vi "NI_controller_Rel_move.vi"(0 "Initialize":bool, 1 "Velocity (10000)":i32=20000 min=-20000000 max=20000000, 4 "Z  rel (mm)":dbl, 5 "Y rel (mm)":dbl, 6 "Motion System":T2=enum."No Motion Card", 7 "X rel (mm)":dbl, 8 "Motion ID":T3=1 min=1 max=32 step=1) -> (12 "Bd ID Out":T1, 14 "X start (mm)":dbl, 15 "Y start (mm)":dbl, 16 "Z start (mm)":dbl, 17 "X Stop (mm)":dbl, 18 "Y Stop (mm)":dbl, 19 "Z Stop (mm)":dbl)   [LabVIEW 2022 SP3]
uses:
  <vilib>/Motion/FlexMotion/CustomControls/CustomControls.llb/AxisOrVectorSpace To Configure.flx
  <vilib>/Motion/FlexMotion/FunctionsVIs/StartStopMotion.llb/Start Motion (8 axes).flx
  -NI_MotionRoutines/MotionSys.ctl
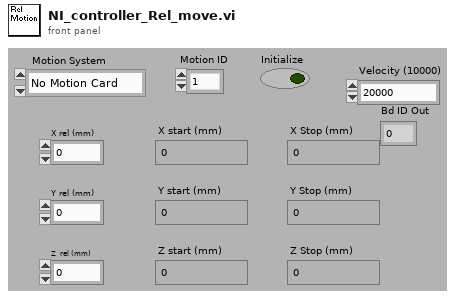
[diagram p1: front panel]
types:
  T1 = typedef "Bd Id Out" = u8
  T2 = typedef "MotionSys.ctl" = enum16{"MM3000", "NI 735x", "Newport ESP", "No Motion Card", "Galil"}
  T3 = typedef "Board Id" = u8
  T4 = enum16{"Absolute Position", "Relative Position", "Velocity", "Relative to Cap Pos", "Modulus Position", "Absolute Contouring", "Relative Contouring"}
  T5 = typedef "AxisOrVectorSpace To Configure.flx" = u16
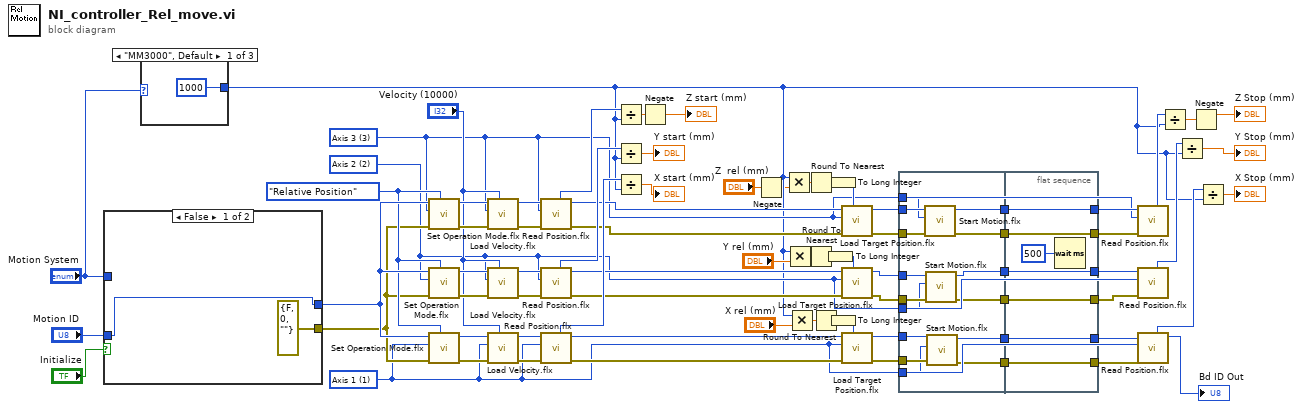
[diagram p0: block diagram]
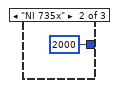
[diagram p2: hidden frame]
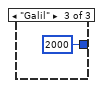
[diagram p3: hidden frame]
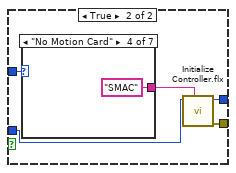
[diagram p4: hidden frame]
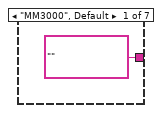
[diagram p5: hidden frame]
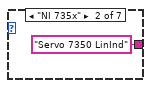
[diagram p6: hidden frame]
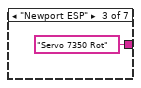
[diagram p7: hidden frame]
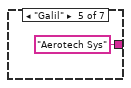
[diagram p8: hidden frame]
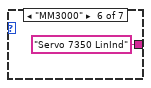
[diagram p9: hidden frame]
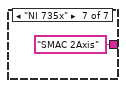
[diagram p10: hidden frame]
diagram:
  w71 = T4."Relative Position" ("Position Mode (Absolute)")
  w18 = T5 3 items=["Axis 1"=1, "Axis 2"=2, "Axis 3"=3, "Axis 4"=4, "Axis 5"=5, "Axis 6"=6, "Axis 7"=7, "Axis 8"=8, "Vector Space 1"=17, "Vector Space 2"=18, "Vector Space 3"=19, "Vector Space 4"=20] ("Axis or Vector Space")
  w19 = T5 2 items=["Axis 1"=1, "Axis 2"=2, "Axis 3"=3, "Axis 4"=4, "Axis 5"=5, "Axis 6"=6, "Axis 7"=7, "Axis 8"=8, "Vector Space 1"=17, "Vector Space 2"=18, "Vector Space 3"=19, "Vector Space 4"=20] ("Axis or Vector Space")
  w17 = T5 1 items=["Axis 1"=1, "Axis 2"=2, "Axis 3"=3, "Axis 4"=4, "Axis 5"=5, "Axis 6"=6, "Axis 7"=7, "Axis 8"=8, "Vector Space 1"=17, "Vector Space 2"=18, "Vector Space 3"=19, "Vector Space 4"=20] ("Axis or Vector Space")
  n1 = case shown="False" "Initialize" {
    tunnel: [w77 w82] -> w72
    tunnel: [errorcluster {"status"=FALSE, "code"=0, "source"=""} ("error out") w81] -> w68
    tunnel: "Motion ID" -> [w77 w79]
    tunnel: "Motion System" -> [_ w78]
    frame False {
    }
    frame True {
      n2 = case shown="\"No Motion Card\"" w78 {
        tunnel: ["" "Servo 7350 LinInd" "Servo 7350 Rot" "SMAC" "Aerotech Sys" "Servo 7350 LinInd" "SMAC 2Axis"] -> w80
        frame "MM3000", Default {
        }
        frame "NI 735x" {
        }
        frame "Newport ESP" {
        }
        frame "No Motion Card" {
        }
        frame "Galil" {
        }
        frame "MM3000" {
        }
        frame "NI 735x" {
        }
      }
      n3 = call <vilib>:"Initialize Controller.flx"("Settings Name"=w80, "Board ID"=w79) -> ("error out"=w81:errorcluster, "Bd ID Out"=w82:T1)  [unwired: 1 in, 5 out]
    }
  }
  n4 = case shown="\"MM3000\", Default" "Motion System" {
    tunnel: [1000 ("y") 2000 ("y") 2000 ("y")] -> w11
    frame "MM3000", Default {
    }
    frame "NI 735x" {
    }
    frame "Galil" {
    }
  }
  n5 = call <vilib>:"Set Operation Mode.flx"("Position Mode (Absolute)"=w71, "error in (no error)"=w68, "Axis or Vector Space"=w18, "Board ID"=w72) -> ("error out"=w67:errorcluster, "Bd ID Out"=w64:T1)  [unwired: 3 out]
  n6 = call <vilib>:"Set Operation Mode.flx"("Position Mode (Absolute)"=w71, "error in (no error)"=w68, "Axis or Vector Space"=w19, "Board ID"=w72) -> ("error out"=w66:errorcluster, "Bd ID Out"=w69:T1)  [unwired: 3 out]
  n7 = call <vilib>:"Set Operation Mode.flx"("Position Mode (Absolute)"=w71, "error in (no error)"=w68, "Axis or Vector Space"=w17, "Board ID"=w72) -> ("error out"=w65:errorcluster, "Bd ID Out"=w70:T1)  [unwired: 3 out]
  n8 = call <vilib>:"Load Velocity.flx"("Velocity (10000)"="Velocity (10000)", "error in (no error)"=w67, "Axis or Vector Space"=w18, "Board ID"=w64) -> ("error out"=w57:errorcluster, "Bd ID Out"=w60:T1)  [unwired: 4 out]
  n9 = call <vilib>:"Load Velocity.flx"("Velocity (10000)"="Velocity (10000)", "error in (no error)"=w66, "Axis or Vector Space"=w19, "Board ID"=w69) -> ("error out"=w58:errorcluster, "Bd ID Out"=w61:T1)  [unwired: 4 out]
  n10 = call <vilib>:"Load Velocity.flx"("Velocity (10000)"="Velocity (10000)", "error in (no error)"=w65, "Axis or Vector Space"=w17, "Board ID"=w70) -> ("error out"=w59:errorcluster, "Bd ID Out"=w62:T1)  [unwired: 4 out]
  n11 = call <vilib>:"Read Position.flx"("error in (no error)"=w57, "Axis"=w18, "Board ID"=w60) -> ("error out"=w47:errorcluster, "Bd ID Out"=w48:T1, "Position"=w54:i32)  [unwired: 4 out]
  n12 = call <vilib>:"Read Position.flx"("error in (no error)"=w58, "Axis"=w19, "Board ID"=w61) -> ("error out"=w46:errorcluster, "Bd ID Out"=w49:T1, "Position"=w55:i32)  [unwired: 4 out]
  n13 = call <vilib>:"Read Position.flx"("error in (no error)"=w59, "Axis"=w17, "Board ID"=w62) -> ("error out"=w45:errorcluster, "Bd ID Out"=w50:T1, "Position"=w56:i32)  [unwired: 4 out]
  n14 = Divide(x=w54, y=w11) -> (x/y=w51:dbl)
  n15 = Divide(x=w55, y=w11) -> (x/y=→"Y start (mm)":dbl)
  n16 = Divide(x=w56, y=w11) -> (x/y=→"X start (mm)":dbl)
  n17 = Negate(x=w51) -> (-x=→"Z start (mm)":dbl)
  n18 = Negate(x="Z  rel (mm)") -> (-x=w10:dbl)
  n19 = Multiply(x=w11, y=w10) -> (x*y=w44:dbl)
  n20 = Multiply(x=w11, y="Y rel (mm)") -> (x*y=w39:dbl)
  n21 = Multiply(x=w11, y="X rel (mm)") -> (x*y=w40:dbl)
  n22 = Round To Nearest(number=w44) -> (nearest integer value=w37:dbl)
  n23 = Round To Nearest(number=w39) -> (nearest integer value=w36:dbl)
  n24 = Round To Nearest(number=w40) -> (nearest integer value=w35:dbl)
  n25 = To Long Integer(number=w36) -> (32bit integer=w33:i32)
  n26 = To Long Integer(number=w37) -> (32bit integer=w34:i32)
  n27 = To Long Integer(number=w35) -> (32bit integer=w32:i32)
  n28 = call <vilib>:"Load Target Position.flx"("Target Position (0)"=w34, "error in (no error)"=w47, "Axis"=w18, "Board ID"=w48) -> ("error out"=w31:errorcluster, "Bd ID Out"=w25:T1)  [unwired: 4 out]
  n29 = call <vilib>:"Load Target Position.flx"("Target Position (0)"=w33, "error in (no error)"=w46, "Axis"=w19, "Board ID"=w49) -> ("error out"=w29:errorcluster, "Bd ID Out"=w23:T1)  [unwired: 4 out]
  n30 = call <vilib>:"Load Target Position.flx"("Target Position (0)"=w32, "error in (no error)"=w45, "Axis"=w17, "Board ID"=w50) -> ("error out"=w27:errorcluster, "Bd ID Out"=w21:T1)  [unwired: 4 out]
  n31 = flat-sequence {
    tunnel: w31 -> [w107]
    tunnel: w29 -> [w105]
    tunnel: w27 -> [w103]
    tunnel: w25 -> [w101]
    tunnel: w23 -> [w99]
    tunnel: w21 -> [w97]
    tunnel: w19 -> [w95]
    tunnel: w18 -> [w94]
    tunnel: w17 -> [w93]
    tunnel: [w106] -> w9
    tunnel: [w104] -> w8
    tunnel: [w102] -> w7
    tunnel: [w100] -> w6
    tunnel: [w98] -> w5
    tunnel: [w96] -> w4
    tunnel: [w109] -> w20
    tunnel: [w110] -> w22
    tunnel: [w111] -> w24
    tunnel: [w112] -> w26
    tunnel: [w113] -> w28
    tunnel: [w114] -> w30
    tunnel: w9 -> [w114]
    tunnel: w8 -> [w113]
    tunnel: w7 -> [w112]
    tunnel: w6 -> [w111]
    tunnel: w5 -> [w110]
    tunnel: w4 -> [w109]
    frame #0 {
      n32 = call-poly <vilib>:"Start Motion.flx"("error in (no error)"=w107, "Axis or Vector Space"=w94, "Board ID"=w101) -> ("error out"=w106:errorcluster, "Bd ID Out"=w100:T1)  [unwired: 1 in, 3 out]
      n33 = call-poly <vilib>:"Start Motion.flx"("error in (no error)"=w105, "Axis or Vector Space"=w95, "Board ID"=w99) -> ("error out"=w104:errorcluster, "Bd ID Out"=w98:T1)  [unwired: 1 in, 3 out]
      n34 = call-poly <vilib>:"Start Motion.flx"("error in (no error)"=w103, "Axis or Vector Space"=w93, "Board ID"=w97) -> ("error out"=w102:errorcluster, "Bd ID Out"=w96:T1)  [unwired: 1 in, 3 out]
    }
    frame #1 {
      n35 = Wait (ms)(milliseconds to wait=u32 500) -> ()  [unwired: 1 out]
    }
  }
  n36 = call <vilib>:"Read Position.flx"("error in (no error)"=w30, "Axis"=w18, "Board ID"=w24) -> ("Position"=w38:i32)  [unwired: 6 out]
  n37 = call <vilib>:"Read Position.flx"("error in (no error)"=w28, "Axis"=w19, "Board ID"=w22) -> ("Position"=w14:i32)  [unwired: 6 out]
  n38 = call <vilib>:"Read Position.flx"("error in (no error)"=w26, "Axis"=w17, "Board ID"=w20) -> ("Bd ID Out"=→"Bd ID Out":T1, "Position"=w12:i32)  [unwired: 5 out]
  n39 = Divide(x=w38, y=w11) -> (x/y=w16:dbl)
  n40 = Divide(x=w14, y=w11) -> (x/y=→"Y Stop (mm)":dbl)
  n41 = Negate(x=w16) -> (-x=→"Z Stop (mm)":dbl)
  n42 = Divide(x=w12, y=w11) -> (x/y=→"X Stop (mm)":dbl)
